vi "Get Checks.vi"(11 "Readiness Report":refnum<class "Readiness Report.lvclass">) -> (3 "Checks":T1[](array[typedef]))   [LabVIEW 2026, in "Readiness Report.lvclass"]
uses:
  Readiness Report.lvclass
  Readiness Report.lvclass/Readiness Report.ctl
  Typedefs/enums/Readiness State Enum.ctl
  Typedefs/clusters/Readiness Check Result.ctl
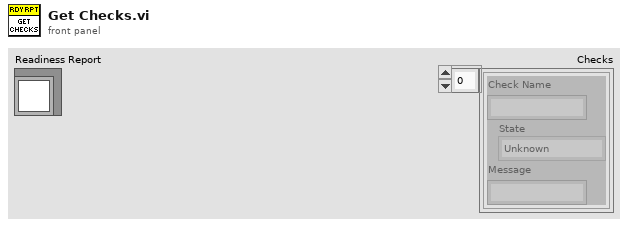
[diagram p1: front panel]
types:
  T1 = typedef "Readiness Check Result.ctl" = cluster{"Check Name":string, "State":T2, "Message":string}
  T2 = typedef "Readiness State Enum.ctl" = enum16{"Unknown", "Ready", "Warning", "NotReady"}
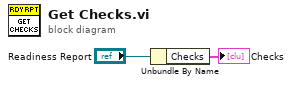
[diagram p0: block diagram]
diagram:
  n1 = Unbundle By Name("Readiness Report") -> ("Checks"=→"Checks":T1[])
